vi "Messdaten_Normieren.vi"(8 "Error In (No Error)":errorcluster, 9 "VISA Name OZ In (OZ)":refnum<visa-resource-name>="USB0::0x0957::0x179B::MY54313507::INSTR", 10 "Oszi-Channel (1)":T1=1.0 min=1.0 max=4.0 step=1.0 format="%#_1g", 11 "Input Array":dbl[](array[numeric])) -> (0 "Error Out":errorcluster, 1 "VISA Name OZ Out":refnum<visa-resource-name>="USB0::0x0957::0x179B::MY54313507::INSTR", 3 "Output Array":dbl[](array[numeric]))   [LabVIEW 2016]
uses:
  Oszi_KanalInfo.ctl
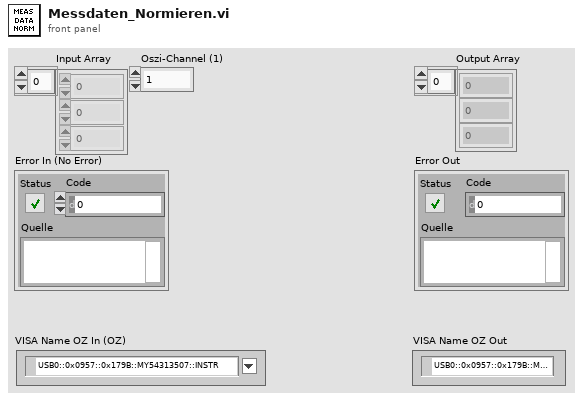
[diagram p1: front panel]
types:
  T1 = typedef "Oszi_KanalInfo.ctl" = dbl
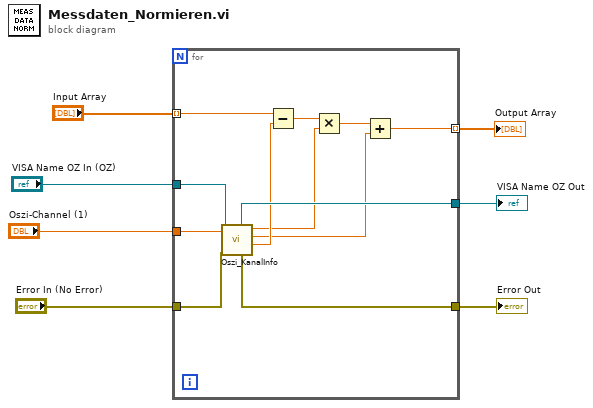
[diagram p0: block diagram]
diagram:
  n1 = for {
    tunnel: "Oszi-Channel (1)" -> [w19]
    tunnel: "VISA Name OZ In (OZ)" -> [w18]
    tunnel: "Error In (No Error)" -> [w17]
    tunnel: [w16] -> w4
    tunnel: [w15] -> w3
    tunnel: "Input Array" -> [w14] mode=indexing
    tunnel: [w8] -> w1 mode=indexing
    n2 = call "Oszi_KanalInfo.vi"("Error In (No Error)"=w17, "Oszi-Channel (1)"=w19, "VISA Name OZ In (OZ)"=w18) -> ("YREFerence"=w13:dbl, "YORigin"=w9:dbl, "YINcrement"=w11:dbl, "Error Out"=w16:errorcluster, "VISA Name OZ Out"=w15:refnum<visa-resource-name>)  [unwired: 3 in, 1 out]
    n3 = Subtract(x=w14, y=w13) -> (x-y=w12:dbl)
    n4 = Multiply(x=w12, y=w11) -> (x*y=w10:dbl)
    n5 = Add(x=w10, y=w9) -> (x+y=w8:dbl)
  }
  "Output Array" <- w1
  "Error Out" <- w4
  "VISA Name OZ Out" <- w3
